vi "SaveStriptestRecoveryFiles.vi"(2 "Arrays format":string, 3 "Array Titles":string, 4 "Strip Segment":string, 5 "no. of arrays":i32, 6 "Actual array lengths":i32, 7 "Region #":u32) -> (0 "Path + Filename OUT":string, 1 "Filename OUT":string)   [LabVIEW 2013]
uses:
  general_VIs/globals/QC_RunInformation.vi
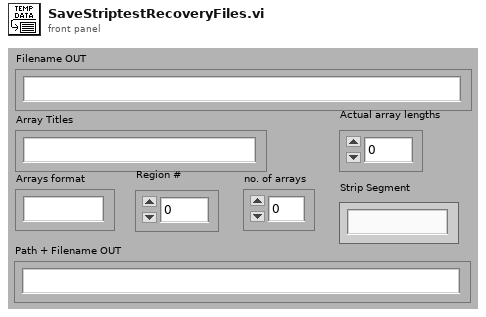
[diagram p1: front panel]
types:
  T1 = enum16{"open", "open or create", "create or replace", "create"}
  T2 = cluster{"Institute":string, "Manufacturers":string[], "Devices":string[], "Serialnumbers Lookup DB":string, "Data directory":string, "Backup & screenshot directory":string, "List of known users":string[]}
  T3 = enum16{"Reset", "Read Array", "Read Element", "Write Element", "Write Array", "Add Element", "Add Array"}
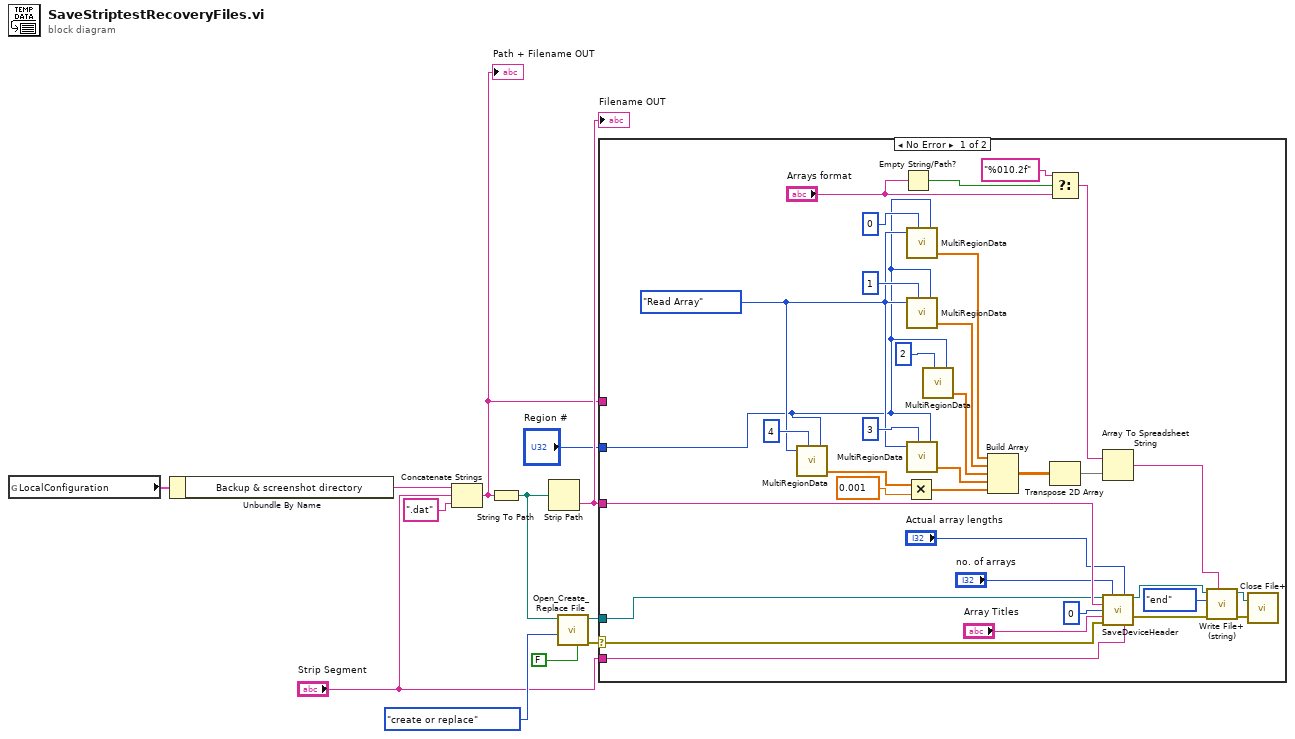
[diagram p0: block diagram]
diagram:
  n1 = global read "QC_RunInformation.vi" "LocalConfiguration"() -> (w4:T2)
  n2 = Unbundle By Name(w4) -> ("Backup & screenshot directory"=w3:string)
  n3 = Concatenate Strings(w3, "Strip Segment", ".dat") -> (w6:string)
  "Path + Filename OUT" <- w6
  n4 = String To Path(string=w6) -> (path=w9:path)
  n5 = Strip Path(path=w9) -> (name=w10:string)  [unwired: 1 out]
  "Filename OUT" <- w10
  n6 = call <vilib>:"Open_Create_Replace File.vi"("advisory dialog? (display:T)"=FALSE, "function (open:0)"=T1."create or replace", "file path"=w9) -> ("error out"=w8:errorcluster, "refnum"=w11:refnum<file>)  [unwired: 5 in, 2 out]
  n7 = case shown="No Error" w8 {
    selector: w8 -> [w46 _]
    tunnel: w11 -> [w43 _]
    tunnel: w6 -> [_ _]
    tunnel: w10 -> [w44 _]
    tunnel: "Region #" -> [w19 _]
    tunnel: "Strip Segment" -> [w14 _]
    frame No Error {
      w28 = T3."Read Array" ("Action")
      n8 = call "MultiRegionData.vi"("Action"=w28, "Array No."=4, "Region index"=w19) -> ("Array OUT"=w26:dbl[])  [unwired: 3 in, 1 out]
      n9 = Empty String/Path?(string/path="Arrays format") -> (empty?=w40:bool)
      n10 = Multiply(x=w26, y=0.001) -> (x*y=w25:dbl[])
      n11 = call "MultiRegionData.vi"("Action"=w28, "Array No."=0, "Region index"=w19) -> ("Array OUT"=w21:dbl[])  [unwired: 3 in, 1 out]
      n12 = call "MultiRegionData.vi"("Action"=w28, "Array No."=1, "Region index"=w19) -> ("Array OUT"=w22:dbl[])  [unwired: 3 in, 1 out]
      n13 = call "MultiRegionData.vi"("Action"=w28, "Array No."=3, "Region index"=w19) -> ("Array OUT"=w24:dbl[])  [unwired: 3 in, 1 out]
      n14 = call "MultiRegionData.vi"("Array No."=2, "Region index"=w19) -> ("Array OUT"=w23:dbl[])  [unwired: 4 in, 1 out]
      n15 = Build Array(w21, w22, w23, w24, w25) -> (w20:dbl[][])
      n16 = Select(t="%010.2f", s=w40, f="Arrays format") -> (s? t:f=w34:string)
      n17 = Transpose 2D Array(2D array=w20) -> (transposed array=w18:dbl[][])
      n18 = Array To Spreadsheet String(array=w18, 3:w34) -> (spreadsheet string=w17:string)  [unwired: 1 in]
      n19 = call "SaveDeviceHeader.vi"("File Refnum in"=w43, "no. of arrays"="no. of arrays", "Array Lengths"="Actual array lengths", "Filename"=w44, "Run Number"=0, "Array Titles"="Array Titles", "error in (no error)"=w46, "Strip Segment"=w14) -> ("File Refnum out"=w16:refnum<file>, "error out"=w15:errorcluster)  [unwired: 5 in, 1 out]
      n20 = call <vilib>:"Write File+ (string).vi"("string"=w17, "error in (no error)"=w15, "pos mode (rel. to end:1)"=enum16{"start", "end", "current"}."end", "refnum"=w16) -> ("error out"=w36:errorcluster, "dup refnum"=w37:refnum<file>)  [unwired: 3 in, 1 out]
      n21 = call <vilib>:"Close File+.vi"("error in (no error)"=w36, "refnum"=w37) -> ()  [unwired: 3 in, 3 out]
    }
    frame Error {
    }
  }
